vi "MP-285 GoTo Position.vi"(0 "VISA resource name":refnum<visa-resource-name>, 1 "Input: Y axis (microns)":dbl format="%.2f", 2 "Input: Z axis (microns)":dbl format="%.2f", 3 "error in (no error)":errorcluster, 4 "Input: X axis (microns)":dbl format="%.2f") -> (5 "VISA resource name out":refnum<visa-resource-name>, 6 "error out":errorcluster)   [LabVIEW 2010]
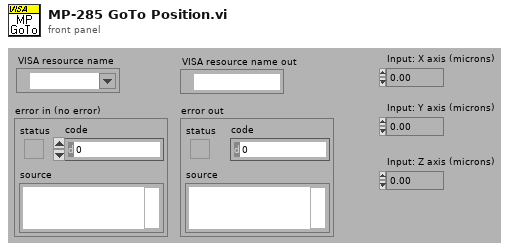
[diagram p1: front panel]
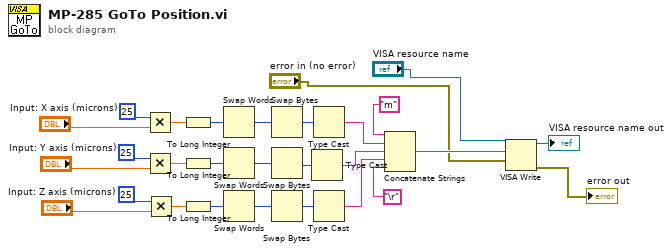
[diagram p0: block diagram]
diagram:
  n1 = Multiply(x=25, y="Input: X axis (microns)") -> (x*y=w18:dbl)
  n2 = Multiply(x=25, y="Input: Y axis (microns)") -> (x*y=w19:dbl)
  n3 = Multiply(x=25, y="Input: Z axis (microns)") -> (x*y=w20:dbl)
  n4 = To Long Integer(number=w18) -> (32bit integer=w21:i32)
  n5 = To Long Integer(number=w19) -> (32bit integer=w25:i32)
  n6 = To Long Integer(number=w20) -> (32bit integer=w26:i32)
  n7 = Swap Words(1:w21) -> (0:w22:i32)
  n8 = Swap Words(1:w25) -> (0:w23:i32)
  n9 = Swap Words(1:w26) -> (0:w24:i32)
  n10 = Swap Bytes(anything=w22) -> (byte swapped=w11:i32)
  n11 = Swap Bytes(anything=w23) -> (byte swapped=w12:i32)
  n12 = Swap Bytes(anything=w24) -> (byte swapped=w13:i32)
  n13 = Type Cast(x=w12) -> (*(type *) &x=w10:string)  [unwired: 1 out]
  n14 = Type Cast(x=w11) -> (*(type *) &x=w8:string)  [unwired: 1 out]
  n15 = Type Cast(x=w13) -> (*(type *) &x=w9:string)  [unwired: 1 out]
  n16 = Concatenate Strings("m", w8, w10, w9, "\r") -> (w6:string)
  n17 = VISA Write(VISA resource name="VISA resource name", write buffer=w6, error in (no error)="error in (no error)") -> (VISA resource name out=→"VISA resource name out":refnum<visa-resource-name>, error out=→"error out":errorcluster)  [unwired: 1 out]
